vi "run_properties.get.vi"(11 "Run in":refnum<class "Run.lvclass">) -> (2 "Run Properties":map{string, string}(c390), 3 "Run out":refnum<class "Run.lvclass">)   [LabVIEW 2020, in "Run.lvclass"]
uses:
  Run.lvclass
  Run.lvclass/Run.ctl
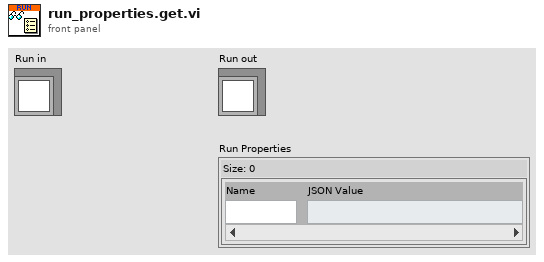
[diagram p1: front panel]
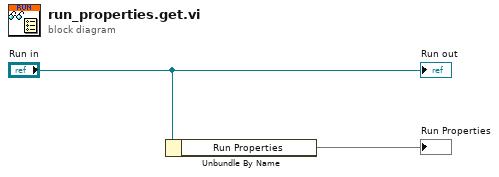
[diagram p0: block diagram]
diagram:
  n1 = Unbundle By Name("Run in") -> ("Run Properties"=→"Run Properties":map{string, string})
  "Run out" <- "Run in"
